vi "xcorr bkp energy.vi"(4 "shift":u8, 5 "Normalization factor":fxp<+,8,1>=1.0, 6 "N":u8, 7 "y":u32, 8 "x":u32, 9 "enable":bool, 10 "lag":u16) -> (1 "Rxy valid":bool, 2 "Rxy":u64, 3 "trigger":bool)   [LabVIEW 2017]
uses:
  <vilib>/rvi/FXPMathLib/FxpDiv/subVIs/nifxpmath_Div_SimConfig.ctl
  <vilib>/rvi/FXPMathLib/FxpDiv/simVIs/DllFxpDivTemp_sub.vi
  <vilib>/rvi/FXPMathLib/FxpDiv/XNode/nifxpmath_Div.xnode
  <vilib>/rvi/FXPMathLib/basic elements/FxpDiscreteDelay/XNode/nifxpmath_DiscreteDelay.xnode
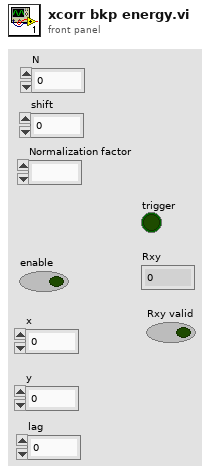
[diagram p1: front panel]
types:
  T1 = cluster{"Q":bool, "Q":bool, "Q":bool, "Q":bool, "valid":bool}
  T2 = cluster{"Q":bool, "Q":bool, "Q":bool, "Q":bool, "Q":bool, "Q":bool, "valid":bool}
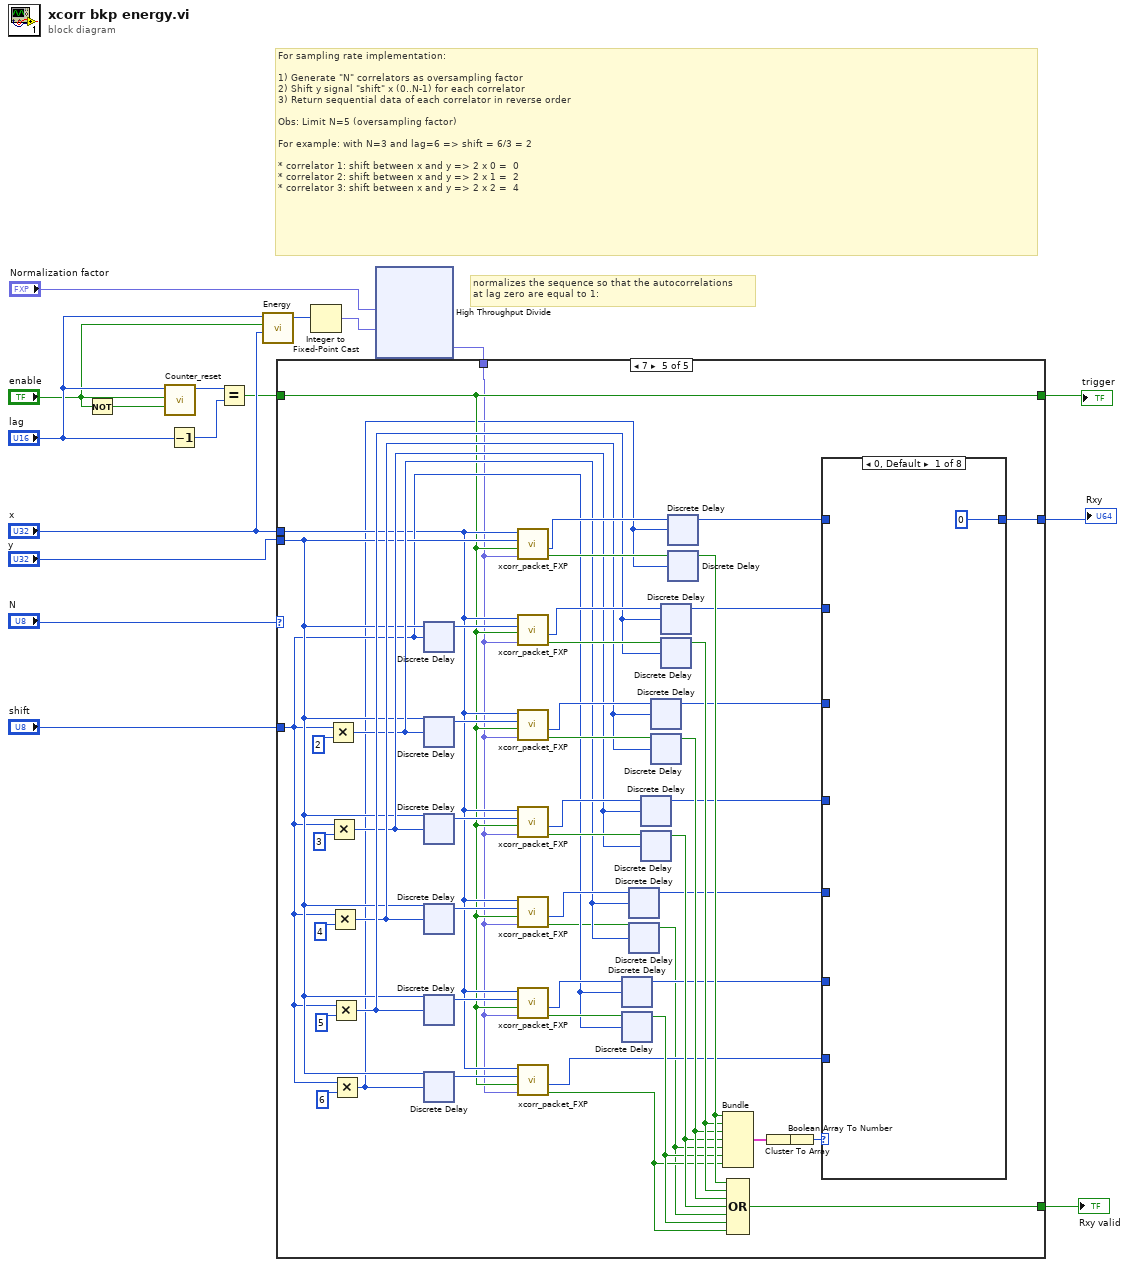
[diagram p0: block diagram]
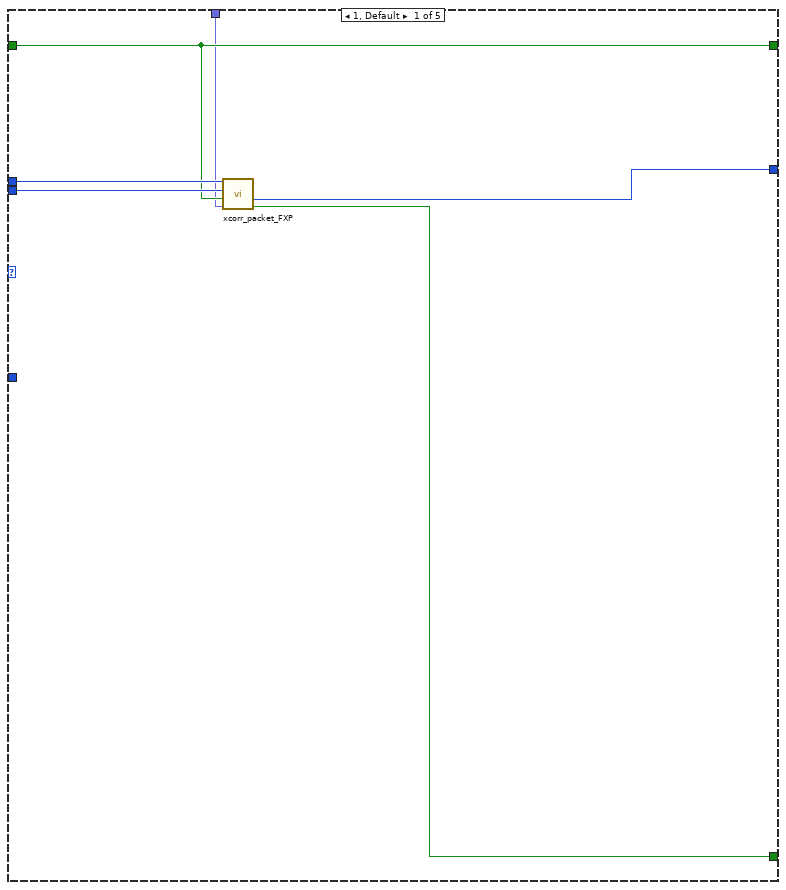
[diagram p2: hidden frame]
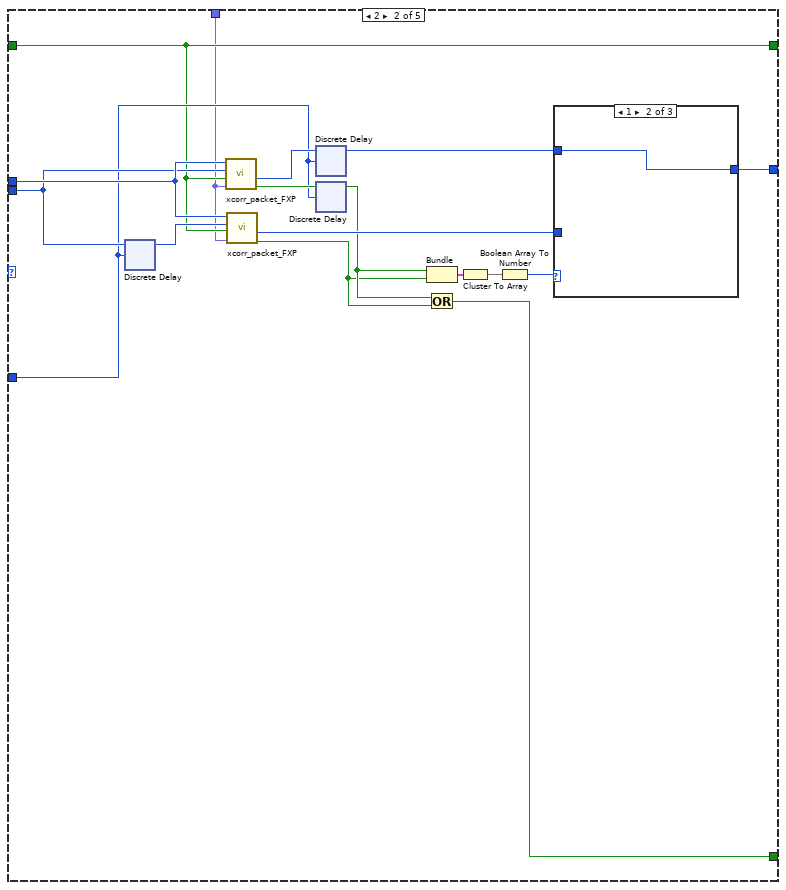
[diagram p3: hidden frame]
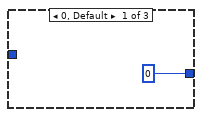
[diagram p4: hidden frame]
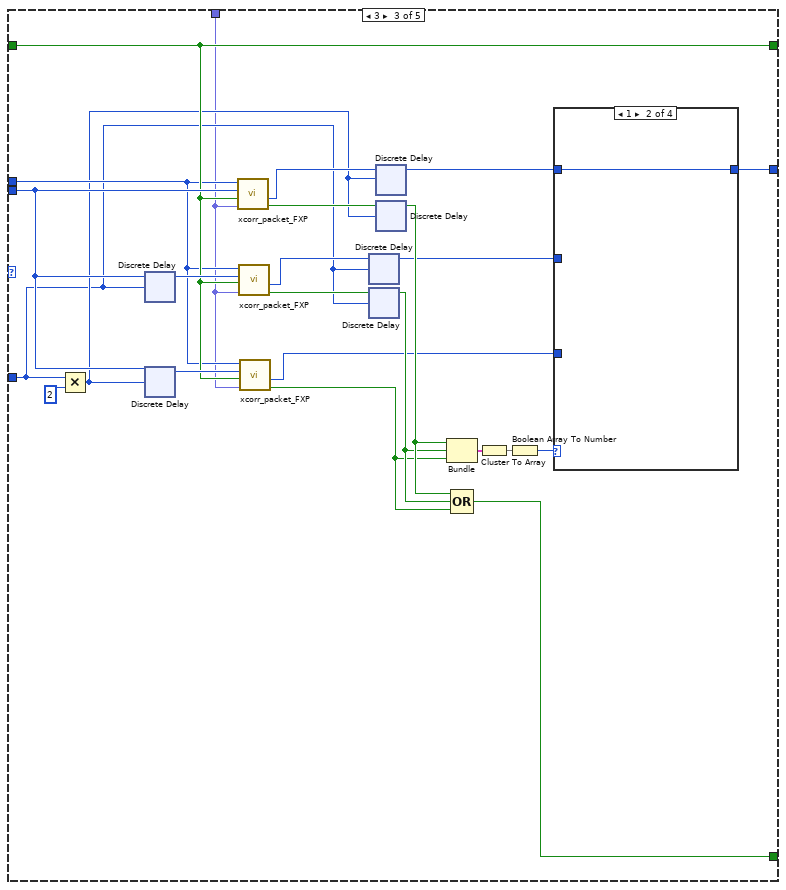
[diagram p6: hidden frame]
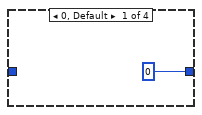
[diagram p7: hidden frame]
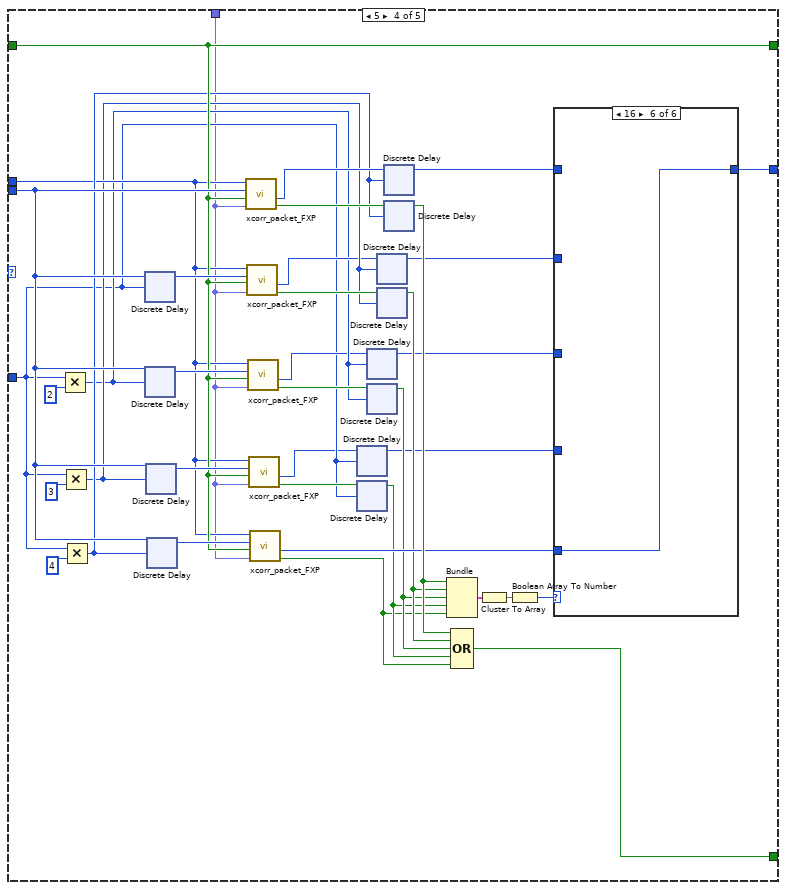
[diagram p10: hidden frame]
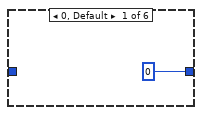
[diagram p11: hidden frame]
diagram:
  # "normalizes the sequence so that the autocorrelations \nat lag zero are equal to 1:"
  # "For sampling rate implementation:\n\n1) Generate \"N\" correlators as oversampling factor\n2) Shift y signal \"shift\" x (0..N-1) for each correlator\n3) Return sequential data of each correlator in reverse order\n\nObs: Limit N=5 (oversampling factor)\n\nFor example: with N=3 and lag=6 => shift = 6/3 = 2\n\n* correlator 1: shift between x and y => 2 x 0 =  0\n* correlator 2: shift between x and y => 2 x 1 =  2\n* correlator 3: shift between x and y => 2 x 2 =  4"
  n1 = Not(x="enable") -> (.not. x?=w14:bool)
  n2 = call "Counter_reset.vi"("reset"=w14, "enable"="enable", "limit"="lag") -> ("count"=w15:u16)  [unwired: 8 in]
  n3 = Decrement(x="lag") -> (x-1=w12:u16)
  n4 = Equal?(x=w15, y=w12) -> (x = y?=w6:bool)
  n5 = call "Energy.vi"("data in"="x", "data in valid"="enable", "Pulse width"="lag") -> ("out"=w4:u32)  [unwired: 7 in, 1 out]
  n6 = Integer to Fixed-Point Cast(integer=w4) -> (fixed-point=w2:fxp<+,32,32>)  [unwired: 1 in]
  n7 = xnode "High Throughput Divide"("x"="Normalization factor", "y"=w2) -> ("x/y"=w1:fxp<+,38,0>)
  n8 = case shown="7" "N" {
    tunnel: [w19 w27 w61 w101 w160] -> w10
    tunnel: [w23 w39 w67 w109 w167] -> w17
    tunnel: [w20 w33 w57 w93 w123] -> w16
    tunnel: w6 -> [w20 w33 w57 w93 w123]
    tunnel: "x" -> [w22 w40 w53 w83 w124]
    tunnel: "y" -> [w21 w38 w58 w94 w126]
    tunnel: "shift" -> [_ w34 w49 w75 w125]
    tunnel: w1 -> [w18 w24 w44 w72 w116]
    frame 1, Default {
      n9 = call "xcorr_packet_FXP.vi"("x"=w22, "y"=w21, "trigger"=w20, "normalization"=w18) -> ("out"=w19:u64, "valid"=w23:bool)  [unwired: 4 in]
    }
    frame 2 {
      n10 = xnode ("Discrete Delay")("D"=w38, "n-1[0..255]"=w34) -> ("Q"=w37:u32)
      n11 = call "xcorr_packet_FXP.vi"("x"=w40, "y"=w38, "trigger"=w33, "normalization"=w24) -> ("out"=w36:u64, "valid"=w35:bool)  [unwired: 4 in]
      n12 = call "xcorr_packet_FXP.vi"("x"=w40, "y"=w37, "trigger"=w33, "normalization"=w24) -> ("out"=w28:u64, "valid"=w25:bool)  [unwired: 4 in]
      n13 = xnode ("Discrete Delay")("D"=w36, "n-1[0..255]"=w34) -> ("Q"=w29:u64)
      n14 = xnode ("Discrete Delay")("D"=w35, "n-1[0..255]"=w34) -> ("Q"=w26:bool)
      n15 = Bundle("Q"=w26, "valid"=w25) -> (w32:cluster{"Q":bool, "valid":bool})  [unwired: 1 in]
      n16 = Or(x=w26, y=w25) -> (x .or. y?=w39:bool)
      n17 = Cluster To Array(cluster=w32) -> (array=w31:bool[])
      n18 = Boolean Array To Number(Boolean array=w31) -> (number=w30:u8)
      n19 = case shown="1" w30 {
        tunnel: [u64 0 ("out") w42 w43] -> w27
        tunnel: w29 -> [_ w42 _]
        tunnel: w28 -> [_ _ w43]
        frame 0, Default {
        }
        frame 1 {
        }
        frame 2 {
        }
      }
    }
    frame 3 {
      n20 = Multiply(x=w49, y=u8 2 ("x")) -> (x*y=w50:u8)
      n21 = xnode ("Discrete Delay")("D"=w58, "n-1[0..255]"=w49) -> ("Q"=w66:u32)
      n22 = xnode ("Discrete Delay")("D"=w58, "n-1[0..255]"=w50) -> ("Q"=w59:u32)
      n23 = call "xcorr_packet_FXP.vi"("x"=w53, "y"=w58, "trigger"=w57, "normalization"=w44) -> ("out"=w65:u64, "valid"=w64:bool)  [unwired: 4 in]
      n24 = call "xcorr_packet_FXP.vi"("x"=w53, "y"=w66, "trigger"=w57, "normalization"=w44) -> ("out"=w52:u64, "valid"=w54:bool)  [unwired: 4 in]
      n25 = call "xcorr_packet_FXP.vi"("x"=w53, "y"=w59, "trigger"=w57, "normalization"=w44) -> ("out"=w45:u64, "valid"=w46:bool)  [unwired: 4 in]
      n26 = xnode ("Discrete Delay")("D"=w52, "n-1[0..255]"=w49) -> ("Q"=w51:u64)
      n27 = xnode ("Discrete Delay")("D"=w54, "n-1[0..255]"=w49) -> ("Q"=w55:bool)
      n28 = xnode ("Discrete Delay")("D"=w65, "n-1[0..255]"=w50) -> ("Q"=w62:u64)
      n29 = xnode ("Discrete Delay")("D"=w64, "n-1[0..255]"=w50) -> ("Q"=w56:bool)
      n30 = Bundle("Q"=w56, "Q"=w55, "valid"=w46) -> (w48:cluster{"Q":bool, "Q":bool, "valid":bool})  [unwired: 1 in]
      n31 = Compound Arithmetic op=OR(w56, w55, w46) -> (w67:bool)
      n32 = Cluster To Array(cluster=w48) -> (array=w47:bool[])
      n33 = Boolean Array To Number(Boolean array=w47) -> (number=w63:u8)
      n34 = case shown="1" w63 {
        tunnel: [u64 0 ("out") w69 w70 w71] -> w61
        tunnel: w62 -> [_ w69 _ _]
        tunnel: w51 -> [_ _ w70 _]
        tunnel: w45 -> [_ _ _ w71]
        frame 0, Default {
        }
        frame 1 {
        }
        frame 2 {
        }
        frame 4 {
        }
      }
    }
    frame 5 {
      n35 = Multiply(x=w75, y=u8 2 ("x")) -> (x*y=w78:u8)
      n36 = Multiply(x=w75, y=u8 3 ("x")) -> (x*y=w81:u8)
      n37 = Multiply(x=w75, y=u8 4 ("x")) -> (x*y=w90:u8)
      n38 = xnode ("Discrete Delay")("D"=w94, "n-1[0..255]"=w75) -> ("Q"=w108:u32)
      n39 = xnode ("Discrete Delay")("D"=w94, "n-1[0..255]"=w78) -> ("Q"=w99:u32)
      n40 = xnode ("Discrete Delay")("D"=w94, "n-1[0..255]"=w81) -> ("Q"=w97:u32)
      n41 = xnode ("Discrete Delay")("D"=w94, "n-1[0..255]"=w90) -> ("Q"=w95:u32)
      n42 = call "xcorr_packet_FXP.vi"("x"=w83, "y"=w94, "trigger"=w93, "normalization"=w72) -> ("out"=w107:u64, "valid"=w106:bool)  [unwired: 4 in]
      n43 = call "xcorr_packet_FXP.vi"("x"=w83, "y"=w108, "trigger"=w93, "normalization"=w72) -> ("out"=w80:u64, "valid"=w88:bool)  [unwired: 4 in]
      n44 = call "xcorr_packet_FXP.vi"("x"=w83, "y"=w99, "trigger"=w93, "normalization"=w72) -> ("out"=w77:u64, "valid"=w87:bool)  [unwired: 4 in]
      n45 = call "xcorr_packet_FXP.vi"("x"=w83, "y"=w97, "trigger"=w93, "normalization"=w72) -> ("out"=w74:u64, "valid"=w85:bool)  [unwired: 4 in]
      n46 = call "xcorr_packet_FXP.vi"("x"=w83, "y"=w95, "trigger"=w93, "normalization"=w72) -> ("out"=w91:u64, "valid"=w82:bool)  [unwired: 4 in]
      n47 = xnode ("Discrete Delay")("D"=w74, "n-1[0..255]"=w75) -> ("Q"=w73:u64)
      n48 = xnode ("Discrete Delay")("D"=w85, "n-1[0..255]"=w75) -> ("Q"=w84:bool)
      n49 = xnode ("Discrete Delay")("D"=w77, "n-1[0..255]"=w78) -> ("Q"=w76:u64)
      n50 = xnode ("Discrete Delay")("D"=w87, "n-1[0..255]"=w78) -> ("Q"=w86:bool)
      n51 = xnode ("Discrete Delay")("D"=w80, "n-1[0..255]"=w81) -> ("Q"=w79:u64)
      n52 = xnode ("Discrete Delay")("D"=w88, "n-1[0..255]"=w81) -> ("Q"=w89:bool)
      n53 = xnode ("Discrete Delay")("D"=w107, "n-1[0..255]"=w90) -> ("Q"=w102:u64)
      n54 = xnode ("Discrete Delay")("D"=w106, "n-1[0..255]"=w90) -> ("Q"=w92:bool)
      n55 = Bundle("Q"=w92, "Q"=w89, "Q"=w86, "Q"=w84, "valid"=w82) -> (w105:T1)  [unwired: 1 in]
      n56 = Compound Arithmetic op=OR(w92, w89, w86, w84, w82) -> (w109:bool)
      n57 = Cluster To Array(cluster=w105) -> (array=w104:bool[])
      n58 = Boolean Array To Number(Boolean array=w104) -> (number=w103:u8)
      n59 = case shown="16" w103 {
        tunnel: [u64 0 ("out") w111 w112 w113 w114 w115] -> w101
        tunnel: w102 -> [_ w111 _ _ _ _]
        tunnel: w79 -> [_ _ w112 _ _ _]
        tunnel: w76 -> [_ _ _ w113 _ _]
        tunnel: w73 -> [_ _ _ _ w114 _]
        tunnel: w91 -> [_ _ _ _ _ w115]
        frame 0, Default {
        }
        frame 1 {
        }
        frame 2 {
        }
        frame 4 {
        }
        frame 8 {
        }
        frame 16 {
        }
      }
    }
    frame 7 {
      n60 = Multiply(x=w125, y=u8 2 ("x")) -> (x*y=w129:u8)
      n61 = Multiply(x=w125, y=u8 3 ("x")) -> (x*y=w130:u8)
      n62 = Multiply(x=w125, y=u8 4 ("x")) -> (x*y=w131:u8)
      n63 = Multiply(x=w125, y=u8 5 ("x")) -> (x*y=w132:u8)
      n64 = Multiply(x=w125, y=u8 6 ("x")) -> (x*y=w120:u8)
      n65 = xnode ("Discrete Delay")("D"=w126, "n-1[0..255]"=w125) -> ("Q"=w166:u32)
      n66 = xnode ("Discrete Delay")("D"=w126, "n-1[0..255]"=w129) -> ("Q"=w158:u32)
      n67 = xnode ("Discrete Delay")("D"=w126, "n-1[0..255]"=w130) -> ("Q"=w156:u32)
      n68 = xnode ("Discrete Delay")("D"=w126, "n-1[0..255]"=w131) -> ("Q"=w154:u32)
      n69 = xnode ("Discrete Delay")("D"=w126, "n-1[0..255]"=w132) -> ("Q"=w139:u32)
      n70 = xnode ("Discrete Delay")("D"=w126, "n-1[0..255]"=w120) -> ("Q"=w127:u32)
      n71 = call "xcorr_packet_FXP.vi"("x"=w124, "y"=w126, "trigger"=w123, "normalization"=w116) -> ("out"=w165:u64, "valid"=w164:bool)  [unwired: 4 in]
      n72 = call "xcorr_packet_FXP.vi"("x"=w124, "y"=w166, "trigger"=w123, "normalization"=w116) -> ("out"=w146:u64, "valid"=w151:bool)  [unwired: 4 in]
      n73 = call "xcorr_packet_FXP.vi"("x"=w124, "y"=w158, "trigger"=w123, "normalization"=w116) -> ("out"=w144:u64, "valid"=w150:bool)  [unwired: 4 in]
      n74 = call "xcorr_packet_FXP.vi"("x"=w124, "y"=w156, "trigger"=w123, "normalization"=w116) -> ("out"=w142:u64, "valid"=w148:bool)  [unwired: 4 in]
      n75 = call "xcorr_packet_FXP.vi"("x"=w124, "y"=w154, "trigger"=w123, "normalization"=w116) -> ("out"=w134:u64, "valid"=w118:bool)  [unwired: 4 in]
      n76 = call "xcorr_packet_FXP.vi"("x"=w124, "y"=w139, "trigger"=w123, "normalization"=w116) -> ("out"=w136:u64, "valid"=w138:bool)  [unwired: 4 in]
      n77 = call "xcorr_packet_FXP.vi"("x"=w124, "y"=w127, "trigger"=w123, "normalization"=w116) -> ("out"=w119:u64, "valid"=w122:bool)  [unwired: 4 in]
      n78 = xnode ("Discrete Delay")("D"=w136, "n-1[0..255]"=w125) -> ("Q"=w135:u64)
      n79 = xnode ("Discrete Delay")("D"=w138, "n-1[0..255]"=w125) -> ("Q"=w137:bool)
      n80 = xnode ("Discrete Delay")("D"=w134, "n-1[0..255]"=w129) -> ("Q"=w133:u64)
      n81 = xnode ("Discrete Delay")("D"=w118, "n-1[0..255]"=w129) -> ("Q"=w117:bool)
      n82 = xnode ("Discrete Delay")("D"=w142, "n-1[0..255]"=w130) -> ("Q"=w141:u64)
      n83 = xnode ("Discrete Delay")("D"=w148, "n-1[0..255]"=w130) -> ("Q"=w147:bool)
      n84 = xnode ("Discrete Delay")("D"=w144, "n-1[0..255]"=w131) -> ("Q"=w143:u64)
      n85 = xnode ("Discrete Delay")("D"=w150, "n-1[0..255]"=w131) -> ("Q"=w149:bool)
      n86 = xnode ("Discrete Delay")("D"=w146, "n-1[0..255]"=w132) -> ("Q"=w145:u64)
      n87 = xnode ("Discrete Delay")("D"=w151, "n-1[0..255]"=w132) -> ("Q"=w152:bool)
      n88 = xnode ("Discrete Delay")("D"=w165, "n-1[0..255]"=w120) -> ("Q"=w161:u64)
      n89 = xnode ("Discrete Delay")("D"=w164, "n-1[0..255]"=w120) -> ("Q"=w153:bool)
      n90 = Bundle("Q"=w153, "Q"=w152, "Q"=w149, "Q"=w147, "Q"=w117, "Q"=w137, "valid"=w122) -> (w121:T2)  [unwired: 1 in]
      n91 = Compound Arithmetic op=OR(w153, w152, w149, w147, w117, w137, w122) -> (w167:bool)
      n92 = Cluster To Array(cluster=w121) -> (array=w163:bool[])
      n93 = Boolean Array To Number(Boolean array=w163) -> (number=w162:u8)
      n94 = case shown="0, Default" w162 {
        tunnel: [u64 0 ("out") w169 w170 w171 w172 w173 w174 w175] -> w160
        tunnel: w161 -> [_ w169 _ _ _ _ _ _]
        tunnel: w145 -> [_ _ w170 _ _ _ _ _]
        tunnel: w143 -> [_ _ _ w171 _ _ _ _]
        tunnel: w141 -> [_ _ _ _ w172 _ _ _]
        tunnel: w133 -> [_ _ _ _ _ w173 _ _]
        tunnel: w135 -> [_ _ _ _ _ _ w174 _]
        tunnel: w119 -> [_ _ _ _ _ _ _ w175]
        frame 0, Default {
        }
        frame 1 {
        }
        frame 2 {
        }
        frame 4 {
        }
        frame 8 {
        }
        frame 16 {
        }
        frame 32 {
        }
        frame 64 {
        }
      }
    }
  }
  "trigger" <- w16
  "Rxy valid" <- w17
  "Rxy" <- w10
